vi "Scratch.vi"() -> ()   [LabVIEW 2019]
uses:
  <vilib>/regexp/Match Regular Expression.xnode
  <vilib>/SLL Toolkit/SLL String/SLL String.lvlib
panel:
  out "Values":string[](array[string])
  in  "Input String":string="This library name is Lab Error UX. This was created in 2026."
  out "Tags[]":string[](array[string])
  in  "Format String":string="This library name is [Tool Name]. This was created in [Year]."
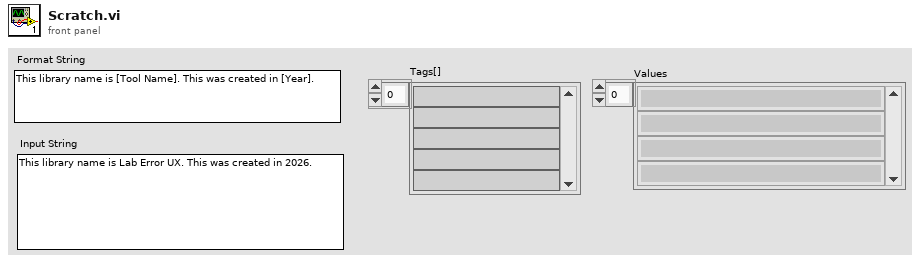
[diagram p1: front panel]
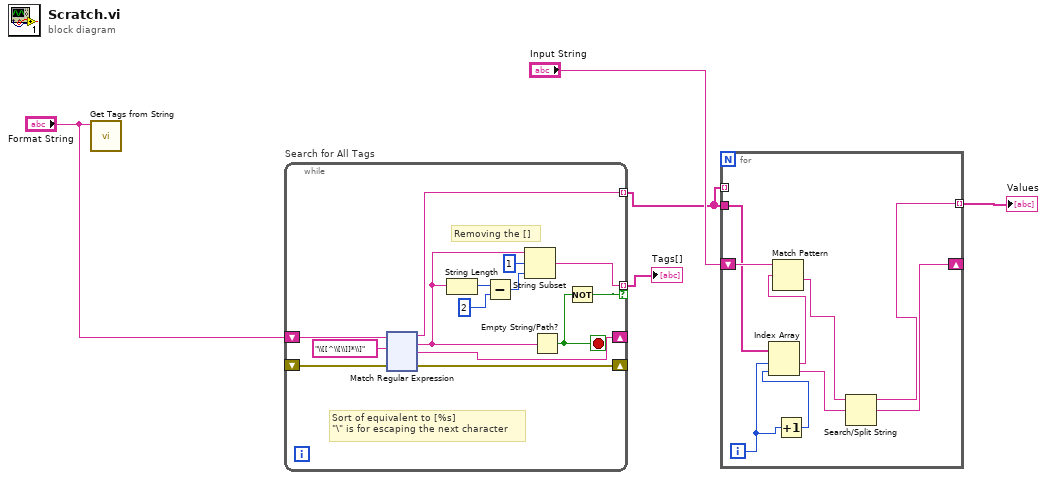
[diagram p0: block diagram]
diagram:
  n1 = call <vilib>:"Get Tags from String.vi"("Input String"="Format String") -> ()  [unwired: 9 in, 2 out]
  n2 = while "Search for All Tags" {
    shift-right: [w17] -> _
    shift-left: _ -> [w18]
    tunnel: [w13] -> w4 mode=indexing if=w14
    tunnel: [w7] -> w1 mode=indexing
    shift-right: [w6] -> _
    shift-left: "Format String" -> [w19]
    stop <- w15 stop-if-true
    # "Removing the []"
    # "Sort of equivalent to [%s]\n\"\\\" is for escaping the next character"
    n3 = xnode "Match Regular Expression"("input string"=w19, "regular expression"="\\[[^\\[\\]]*\\]", "error in"=w18) -> ("before match"=w7:string, "whole match"=w11:string, "after match"=w6:string, "error out"=w17:errorcluster)  [unwired: 3 in, 1 out]
    n4 = String Length(string=w11) -> (length=w10:i32)
    n5 = Subtract(x=w10, y=2) -> (x-y=w8:i32)
    n6 = String Subset(string=w11, offset (0)=1, length (rest)=w8) -> (substring=w13:string)
    n7 = Empty String/Path?(string/path=w11) -> (empty?=w15:bool)
    n8 = Not(x=w15) -> (.not. x?=w14:bool)
  }
  "Tags[]" <- w4
  n9 = for {
    tunnel: w1 -> [w144]
    shift-right: [w138] -> _
    shift-left: "Input String" -> [w145]
    tunnel: [w137] -> w2 mode=indexing
    tunnel: w1 -> [_] mode=indexing
    i -> [w143]
    n10 = Increment(x=w143) -> (x+1=w142:i32)
    n11 = Index Array(array=w144, index #1=w143, index #2=w142) -> (element #1=w141:string, element #2=w139:string)
    n12 = Match Pattern(string=w145, regular expression=w141) -> (after substring=w140:string)  [unwired: 1 in, 3 out]
    n13 = Search/Split String(string=w140, search string/char (-)=w139) -> (substring before match=w137:string, match + rest of string=w138:string)  [unwired: 1 in, 1 out]
  }
  "Values" <- w2
